vi "Move For Time.vi"(8 "error in (no error)":errorcluster, 9 "Time (ms)":u32, 10 "Speed":dbl, 11 "arm.lvclass":refnum<class "arm.lvclass">) -> (0 "error out":errorcluster, 3 "arm.lvclass":refnum<class "arm.lvclass">)   [LabVIEW 2015, in "arm.lvclass"]
uses:
  arm.lvclass
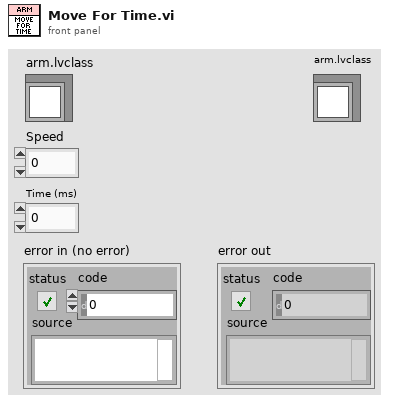
[diagram p1: front panel]
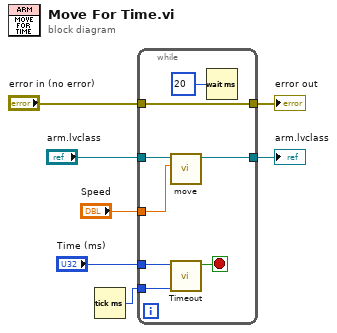
[diagram p0: block diagram]
diagram:
  n1 = Tick Count (ms)() -> (millisecond timer value=w4:u32)
  n2 = while {
    tunnel: "arm.lvclass" -> [w11]
    tunnel: [w12] -> w5
    tunnel: w4 -> [w14]
    tunnel: "Speed" -> [w10]
    tunnel: "Time (ms)" -> [w9]
    tunnel: "error in (no error)" -> [w8]
    tunnel: [w8] -> w1
    stop <- w13 stop-if-true
    n3 = call "move.vi"("Speed"=w10, "arm.lvclass"=w11) -> ("arm.lvclass"=w12:refnum<class "arm.lvclass">)  [unwired: 9 in]
    n4 = call "Timeout.vi"("Start Time In"=w14, "Time Limit"=w9) -> ("Timeout"=w13:bool)  [unwired: 8 in, 1 out]
    n5 = Wait (ms)(milliseconds to wait=u32 20) -> ()  [unwired: 1 out]
  }
  "arm.lvclass" <- w5
  "error out" <- w1
